vi "configuration UI.vi"() -> ()   [LabVIEW 2013, in "CVT editor node.lvclass"]
uses:
  CVT editor node.lvclass
  <vilib>/CEF_TreeControl/Node/NodeRef.ctl
  <vilib>/CEF_TreeControl/Node/NISE_CEF_Node.lvclass
  <vilib>/NI/AMC/Message Queue.ctl
  <vilib>/NI/AMC/Message.ctl
  <vilib>/NI/Tools/Keyed Array/KeyedArray.ctl
  <vilib>/CEF_TreeControl/Node/UserEventRef.ctl
  <vilib>/CEF_TreeControl/Controls/EventCluster.ctl
  <vilib>/NI/Tag Bus Data Framework/Configuration Editor/Classes/Engine Parent/Engine Parent Editor Node.lvclass
  <vilib>/NI/Tag Bus/tag/tag descriptor.lvclass
  <vilib>/NI/Tag Bus/tag/Data Type.ctl
  <vilib>/NI/TBM Modules/CVT Access/module/configuration/CVT configuration.lvclass
  <vilib>/NI/Module Execution Interface/Engine Configuration/engine configuration.lvclass
  <vilib>/NI/Tag Bus/tag/tag descriptor.lvclass/tag descriptor.ctl
  CVT editor node.lvclass/CVT editor node.ctl
  <vilib>/NI/Tag Bus Module Framework/channel/channel classification.ctl
  <vilib>/NI/Tag Bus Module Framework/root configuration/TBM configuration.lvclass/TBM configuration.ctl
  <vilib>/NI/Tag Bus/tag/write tag name.vi
  <vilib>/NI/Tag Bus/tag/write data type.vi
  <vilib>/NI/Tag Bus Module Framework/root configuration/create GUID.vi
  <vilib>/NI/Tag Bus Data Framework/Configuration Editor/Classes/Module editor node/module editor node.lvclass
  <vilib>/CEF_TreeControl/NISE_CEF_TreeControl.lvlib
  <vilib>/NI/Tag Bus Module Framework/channel/TBM channel.lvclass
  <vilib>/NI/Tag Bus Module Framework/root configuration/TBM configuration.lvclass
  <vilib>/NI/Tools/Keyed Array/Tools_KeyedArray.lvlib
  <vilib>/NI/AMC/AMC.lvlib
panel:
  in  "Tab Control":enum32{"Channel Mapping"}(tab)
  in  "Direction":enum32{"From CVT", "To CVT"}(radio)
  in  "remove to":bool
  in  "add to":bool
  in  "remove from":bool
  in  "add from":bool
  in  "toCVTlist":i32(listbox)
  in  "fromCVTlist":i32(listbox)
  in  "avail tags":i32(listbox)=-1
  in  "user event":T1
  in  "main queue":T2
  in  "node ref":T3
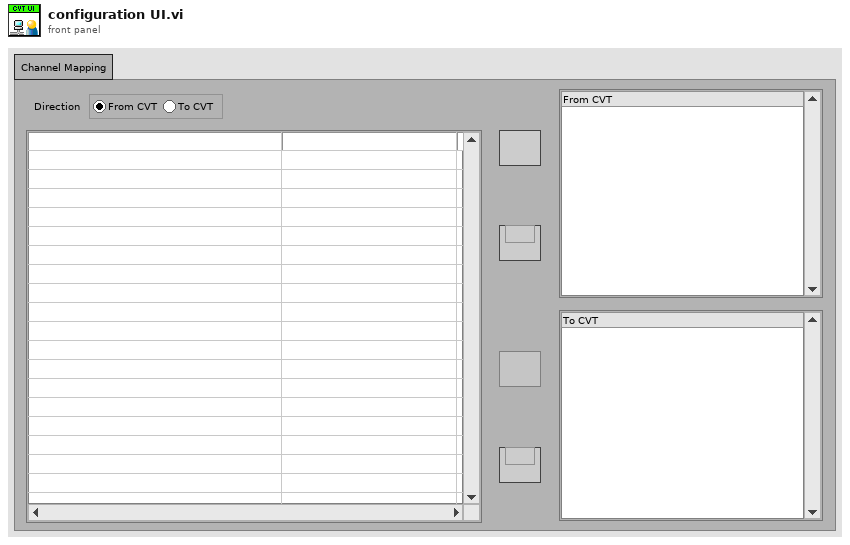
[diagram p1: front panel]
types:
  T1 = typedef "NISE_CEF_Node.lvclass/UserEventRef.ctl" = refnum<user-event>
  T2 = typedef "AMC.lvlib/Message Queue.ctl" = refnum<queue>
  T3 = typedef "NISE_CEF_Node.lvclass/NodeRef.ctl" = refnum<data-value>
  T4 = typedef "NISE_CEF_TreeControl.lvlib/EventCluster.ctl" = cluster{"command":string, "data":string}
  T5 = typedef "tag bus.lvlib/tag descriptor.lvclass/Data Type.ctl" = enum16{"Double", "Single", "I64", "I32", "I16", "I8", "U64", "U32", "U16", "U8", "Boolean", "String", "Array of Double", "Array of Single", "Array of I64", "Array of I32", "Array of I16", "Array of I8", "Array of U64", "Array of U32", "Array of U16", "Array of U8", "Array of Boolean", "Array of String"}
  T6 = enum8{"Enabled", "Disabled", "Disabled and Grayed Out"}
  T7 = typedef "TBM channel.lvclass/channel classification.ctl" = enum16{"input data", "output data", "processing parameter", "processing result"}
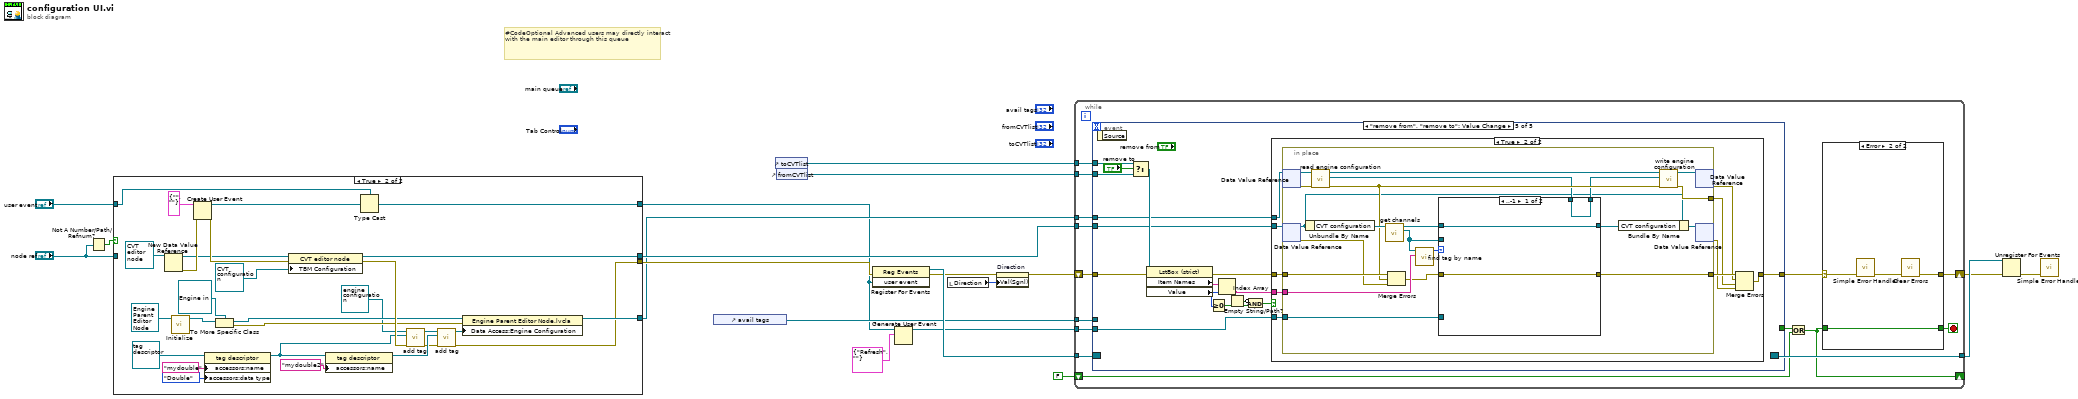
[diagram p0: block diagram]
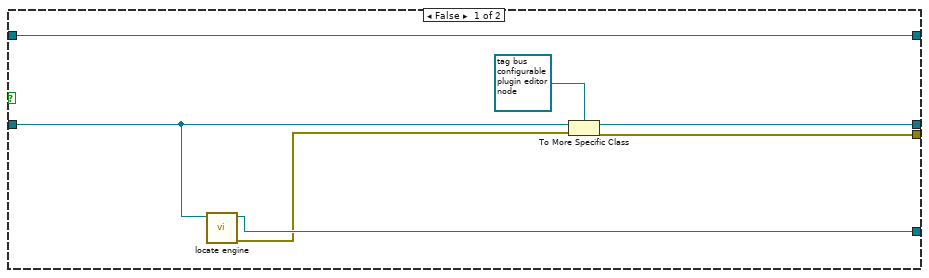
[diagram p2: hidden frame]
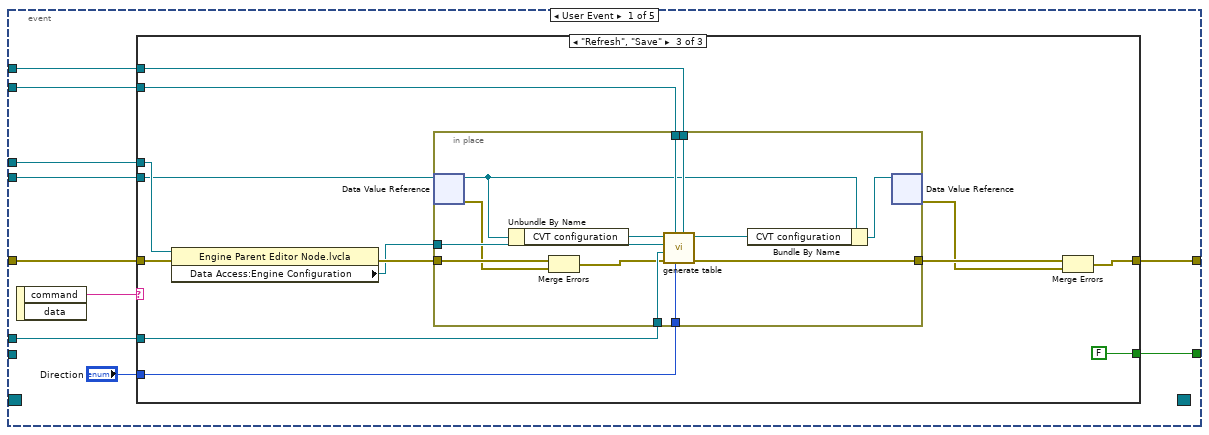
[diagram p4: hidden frame]
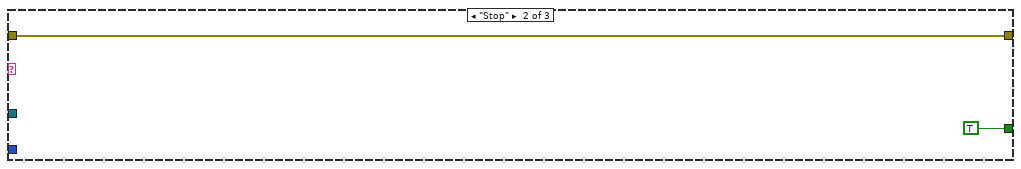
[diagram p6: hidden frame]
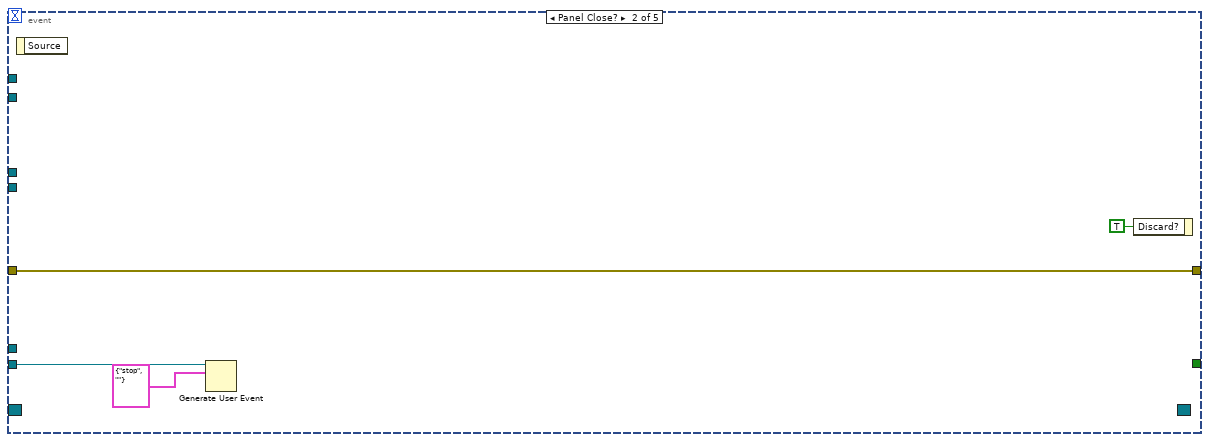
[diagram p7: hidden frame]
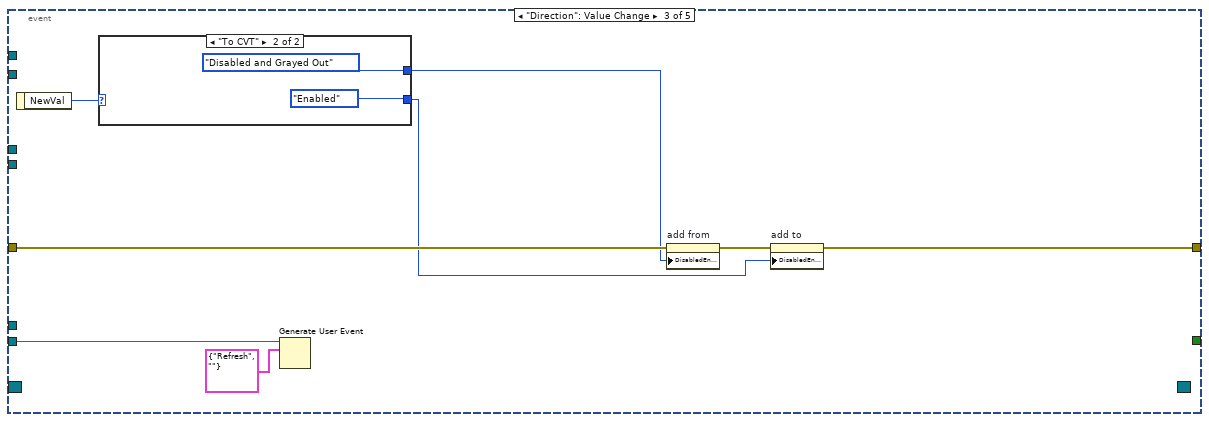
[diagram p8: hidden frame]
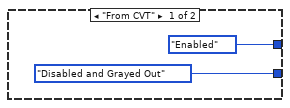
[diagram p9: hidden frame]
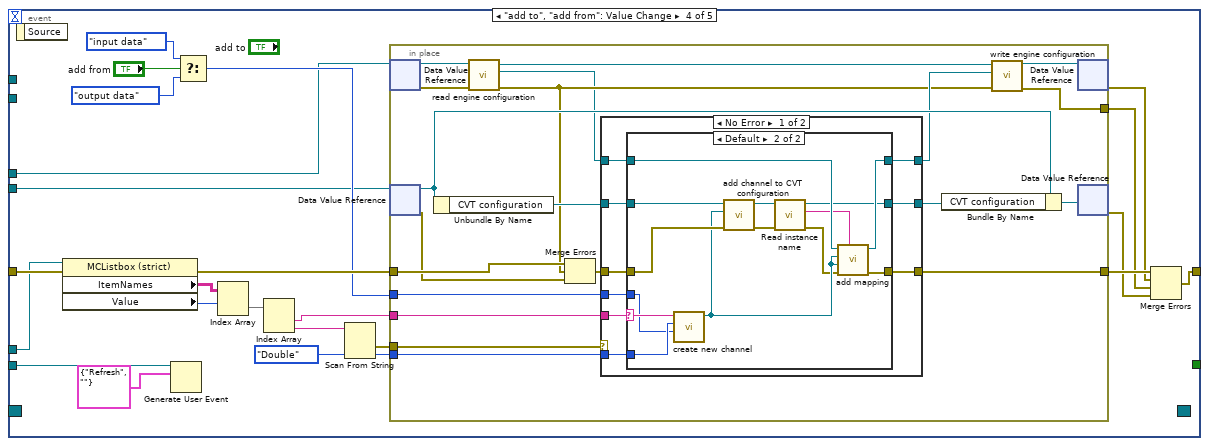
[diagram p10: hidden frame]
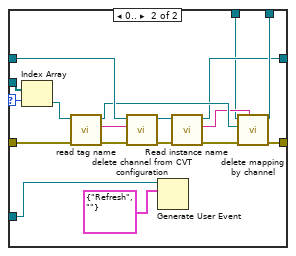
[diagram p14: hidden frame]
diagram:
  # "#CodeOptional Advanced users may directly interact with the main editor through this queue"
  n1 = Not A Number/Path/Refnum?(number/path/refnum="node ref") -> (NaN/Path/Refnum?=w16:bool)
  n2 = case shown="True" w16 {
    tunnel: "user event" -> [w27 w32]
    tunnel: [w27 w33] -> w1
    tunnel: "node ref" -> [w25 _]
    tunnel: [w24 w51] -> w13
    tunnel: [w23 w42] -> w12
    tunnel: [w22 w48] -> w10
    frame False {
      n3 = call <vilib>:"locate engine.vi"("component"=w25) -> ("error out"=w21:errorcluster, "engine"=w22:refnum<data-value>)  [unwired: 9 in]
      n4 = To More Specific Class(target class=refnum<data-value> refnum ("data value reference"), reference=w25, error in=w21) -> (specific class reference=w24:refnum<data-value>, error out=w23:errorcluster)
    }
    frame True {
      n5 = New Data Value Reference(data value=refnum<class "CVT editor node.lvclass"> refnum ("tag bus configurable plugin editor node")) -> (data value reference=w50:refnum<data-value>, error out=w53:errorcluster)  [unwired: 1 in]
      n6 = call-dynamic "Initialize.vi"("Engine in"=refnum<class "Engine Parent Editor Node.lvclass"> refnum) -> ("data value reference"=w37:T3)  [unwired: 8 in, 2 out]
      n7 = Create User Event(user event datatype=T4 {"command"="", "data"=""} ("event data"), error in=w53) -> (user event=w54:refnum<user-event>, error out=w52:errorcluster)
      n8 = property class="tag descriptor"(reference=refnum<class "tag descriptor.lvclass"> refnum ("tag descriptor"), "accessors:name"="mydouble" ("name"), "accessors:data type"=Data_Type."Double" ("data type")) -> (reference out=w40:refnum<class "tag descriptor.lvclass">)  [unwired: 1 in, 1 out]
      n9 = To More Specific Class(target class=refnum<data-value> refnum ("data value reference"), reference=w37) -> (specific class reference=w36:refnum<data-value>, error out=w34:errorcluster)  [unwired: 1 in]
      n10 = property class="CVT editor node"(reference=w50, error in=w52, "TBM Configuration"=refnum<class "CVT configuration.lvclass"> refnum ("CVT configuration")) -> (reference out=w51:refnum<data-value>, error out=w44:errorcluster)
      n11 = property class="tag descriptor"(reference=w40, "accessors:name"="mydouble2" ("name")) -> (reference out=w41:refnum<class "tag descriptor.lvclass">)  [unwired: 1 in, 1 out]
      n12 = Type Cast(type=w32, x=w54) -> (*(type *) &x=w33:T1)
      n13 = call <vilib>:"add tag.vi"("error in"=w44, "tag descriptor"=w40, "engine configuration in"=refnum<class "engine configuration.lvclass"> refnum) -> ("error out"=w31:errorcluster, "engine configuration out"=w30:refnum<class "engine configuration.lvclass">)  [unwired: 7 in]
      n14 = call <vilib>:"add tag.vi"("error in"=w31, "tag descriptor"=w41, "engine configuration in"=w30) -> ("error out"=w42:errorcluster, "engine configuration out"=w29:refnum<class "engine configuration.lvclass">)  [unwired: 7 in]
      n15 = property class="Engine Parent Editor Node.lvcla"(reference=w36, error in=w34, "Data Access:Engine Configuration"=w29) -> (reference out=w48:refnum<data-value>)  [unwired: 1 out]
    }
  }
  n16 = control-ref of="avail tags"() -> (w9:refnum<vi>)
  n17 = control-ref of="toCVTlist"() -> (w8:refnum<vi>)
  n18 = control-ref of="fromCVTlist"() -> (w7:refnum<vi>)
  n19 = register-events(error in=w12, w1) -> (reference out=w20:refnum<event-registration>, error out=w6:errorcluster)  [unwired: 1 in]
  n20 = Generate User Event(user event=w1, event data cluster=T4 {"command"="Refresh", "data"=""} ("event data")) -> (user event out=w2:T1)  [unwired: 2 in, 1 out]
  n21 = local read "Direction"() -> (w4:enum32{"From CVT", "To CVT"})
  n22 = property on="Direction" class="RadioBtnsControl (strict)"(error in=w6, "Val(Sgnl)"=w4) -> (error out=w5:errorcluster)  [unwired: 1 in, 1 out]
  n23 = while {
    tunnel: w20 -> [w70]
    tunnel: [w69] -> w19
    shift-right: [w62] -> w18
    shift-left: w5 -> [w68]
    shift-right: [w64] -> _
    shift-left: FALSE -> [w63]
    tunnel: w13 -> [w61]
    tunnel: w10 -> [w60]
    tunnel: w2 -> [w59]
    tunnel: w9 -> [w58]
    tunnel: w8 -> [w57]
    tunnel: w7 -> [w56]
    stop <- w66 stop-if-true
    n24 = event shown="[4] \"remove from\", \"remove to\": Value Change" {
      selector: w70 -> [_ _ _ _ _]
      dyn-events: [_ _ _ _ _] -> w69
      timeout: _ -> [_ _ _ _ _]
      tunnel: [w86 _ _ _ _] -> w65
      tunnel: [w83 w119 w123 w137 w209] -> w67
      tunnel: w68 -> [w84 w119 w125 w155 w217]
      tunnel: w61 -> [w82 _ _ w133 w206]
      tunnel: w60 -> [w81 _ _ w134 w205]
      tunnel: w59 -> [_ w116 w126 w153 w208]
      tunnel: w58 -> [w80 _ _ w147 _]
      tunnel: w57 -> [w79 _ _ _ w219]
      tunnel: w56 -> [w78 _ _ _ w220]
      event User Event {
        n25 = event-data() -> ("command"=w85:string)  [unwired: 1 in, 1 out]
        n26 = case shown="\"Refresh\", \"Save\"" w85 {
          tunnel: [_ TRUE FALSE] -> w86
          tunnel: w84 -> [w87 w88 w101]
          tunnel: [w87 w88 w91] -> w83
          tunnel: w82 -> [_ _ w92]
          tunnel: w81 -> [_ _ w94]
          tunnel: w80 -> [_ _ w99]
          tunnel: w79 -> [_ _ w98]
          tunnel: w78 -> [_ _ w97]
          tunnel: "Direction" -> [_ _ w96]
          frame Default {
          }
          frame "Stop" {
          }
          frame "Refresh", "Save" {
            n27 = property class="Engine Parent Editor Node.lvcla"(reference=w94, error in=w101) -> (error out=w95:errorcluster, "Data Access:Engine Configuration"=w93:refnum<class "engine configuration.lvclass">)  [unwired: 1 out]
            n28 = in-place {
              in-place-border: [w115] -> w100
              in-place-border: w99 -> [w114]
              in-place-border: w98 -> [w113]
              in-place-border: w97 -> [w112]
              in-place-border: w96 -> [w111]
              in-place-border: w95 -> [w110]
              in-place-border: w93 -> [w109]
              n29 = in-place-dvr #1(w92) -> (w105:refnum<class "CVT editor node.lvclass">, w107:errorcluster)
              n30 = Unbundle By Name(w105) -> ("CVT configuration"=w106:refnum<class "CVT configuration.lvclass">)
              n31 = Merge Errors(w110, w107) -> (w108:errorcluster)
              n32 = call "generate table.vi"("to cvt"=w113, "Direction"=w111, "from cvt"=w112, "error in"=w108, "avail tags"=w114, "engine configuration in"=w109, "cvt in"=w106) -> ("error out"=w115:errorcluster, "cvt out"=w103:refnum<class "CVT configuration.lvclass">)  [unwired: 3 in]
              n33 = Bundle By Name(cluster=w105, "CVT configuration"=w103) -> (w104:refnum<class "CVT editor node.lvclass">)
              n34 = in-place-dvr #1(w104) -> (w90:errorcluster)  [unwired: 1 out]
            }
            n35 = Merge Errors(w100, w90) -> (w91:errorcluster)
          }
        }
      }
      event Panel Close? {
        n36 = event-data() -> ()  [unwired: 1 in, 1 out]
        n37 = Generate User Event(user event=w116, event data cluster=T4 {"command"="stop", "data"=""} ("event data")) -> ()  [unwired: 2 in, 2 out]
        n38 = event-data("Discard?"=TRUE) -> ()  [unwired: 1 in, 1 out]
      }
      event "Direction": Value Change {
        n39 = event-data() -> ("NewVal"=w122:enum32{"From CVT", "To CVT"})  [unwired: 1 in]
        n40 = case shown="\"To CVT\"" w122 {
          tunnel: [T6."Enabled" ("Disabled") T6."Disabled and Grayed Out" ("Disabled")] -> w121
          tunnel: [T6."Disabled and Grayed Out" ("Disabled") T6."Enabled" ("Disabled")] -> w120
          frame "From CVT" {
          }
          frame "To CVT" {
          }
        }
        n41 = Generate User Event(user event=w126, event data cluster=T4 {"command"="Refresh", "data"=""} ("event data")) -> ()  [unwired: 2 in, 2 out]
        n42 = property on="add from" class="Bool"(error in=w125, "DisabledEnum"=w121) -> (error out=w124:errorcluster)  [unwired: 1 in, 1 out]
        n43 = property on="add to" class="Bool"(error in=w124, "DisabledEnum"=w120) -> (error out=w123:errorcluster)  [unwired: 1 in, 1 out]
      }
      event "add to", "add from": Value Change {
        n44 = event-data() -> ()  [unwired: 1 in, 1 out]
        n45 = property class="MCListbox (strict)"(reference=w147, error in=w155) -> (error out=w148:errorcluster, "ItemNames"=w146:string[][], "Value"=w145:i32)  [unwired: 1 out]
        n46 = Generate User Event(user event=w153, event data cluster=T4 {"command"="Refresh", "data"=""} ("event data")) -> ()  [unwired: 2 in, 2 out]
        n47 = Select(t=channel_classification."input data" ("channel classification"), s="add from", f=channel_classification."output data" ("channel classification")) -> (s? t:f=w138:T7)
        n48 = Index Array(array=w146, index (row)=w145) -> (element=w142:string[])  [unwired: 1 in]
        n49 = Index Array(array=w142) -> (element #1=w141:string, element #2=w144:string)  [unwired: 2 in]
        n50 = Scan From String(input string=w144, default 1=Data_Type."Double" ("data type")) -> (error out=w140:errorcluster, output 1=w139:T5)  [unwired: 3 in, 2 out]
        n51 = in-place {
          in-place-border: [w175] -> w154
          in-place-border: w148 -> [w174]
          in-place-border: w141 -> [w173]
          in-place-border: w140 -> [w172]
          in-place-border: w139 -> [w171]
          in-place-border: w138 -> [w170]
          in-place-border: [w160] -> w132
          n52 = in-place-dvr #2(w134) -> (w163:refnum<class "Engine Parent Editor Node.lvclass">, w158:errorcluster)
          n53 = in-place-dvr #3(w133) -> (w166:refnum<class "CVT editor node.lvclass">, w164:errorcluster)
          n54 = Unbundle By Name(w166) -> ("CVT configuration"=w168:refnum<class "CVT configuration.lvclass">)
          n55 = call <vilib>:"read engine configuration.vi"("error in"=w158, "Engine Parent Editor Node in"=w163) -> ("error out"=w157:errorcluster, "engine configuration"=w156:refnum<class "engine configuration.lvclass">, "Engine Parent Editor Node out"=w159:refnum<class "Engine Parent Editor Node.lvclass">)  [unwired: 7 in]
          n56 = Merge Errors(w174, w157, w164) -> (w169:errorcluster)
          n57 = case shown="No Error" w172 {
            tunnel: [w184 w202] -> w175
            tunnel: [w183 w204] -> w161
            tunnel: [w182 w203] -> w167
            tunnel: w168 -> [w181 w203]
            tunnel: w156 -> [w180 w204]
            tunnel: w169 -> [w179 w202]
            tunnel: w173 -> [w178 _]
            tunnel: w171 -> [w177 _]
            tunnel: w170 -> [w176 _]
            frame No Error {
              n58 = case shown="Default" w178 {
                selector: w178 -> [_ w195]
                tunnel: [w187 w201] -> w184
                tunnel: w179 -> [w187 w197]
                tunnel: w180 -> [w185 w200]
                tunnel: [w186 w189] -> w182
                tunnel: w181 -> [w186 w198]
                tunnel: [w185 w199] -> w183
                tunnel: w177 -> [_ w194]
                tunnel: w176 -> [_ w193]
                frame "" {
                }
                frame Default {
                  n59 = call <vilib>:"create new channel.vi"("channel classification"=w193, "data type"=w194, "channel name"=w195) -> ("channel"=w192:refnum<class "TBM channel.lvclass">)  [unwired: 8 in]
                  n60 = call <vilib>:"add channel to CVT configuration.vi"("error in"=w197, "channel"=w192, "CVT configuration in"=w198) -> ("error out"=w196:errorcluster, "CVT configuration out"=w190:refnum<class "CVT configuration.lvclass">)  [unwired: 7 in]
                  n61 = call <vilib>:"Read instance name.vi"("error in"=w196, "configuration in"=w190) -> ("error out"=w191:errorcluster, "instance id"=w188:string, "configuration out"=w189:refnum<class "CVT configuration.lvclass">)  [unwired: 7 in]
                  n62 = call <vilib>:"add mapping.vi"("owner ID"=w188, "error in"=w191, "channel"=w192, "tag descriptor"=w192, "engine configuration"=w200) -> ("error out"=w201:errorcluster, "engine configuration out"=w199:refnum<class "engine configuration.lvclass">)  [unwired: 5 in]
                }
              }
            }
            frame Error {
            }
          }
          n63 = Bundle By Name(cluster=w166, "CVT configuration"=w167) -> (w165:refnum<class "CVT editor node.lvclass">)
          n64 = call <vilib>:"write engine configuration.vi"("error in"=w157, "engine configuration"=w161, "Engine Parent Editor Node in"=w159) -> ("error out"=w160:errorcluster, "Engine Parent Editor Node out"=w162:refnum<class "Engine Parent Editor Node.lvclass">)  [unwired: 7 in]
          n65 = in-place-dvr #2(w162) -> (w136:errorcluster)  [unwired: 1 out]
          n66 = in-place-dvr #3(w165) -> (w135:errorcluster)  [unwired: 1 out]
        }
        n67 = Merge Errors(w154, w136, w132, w135) -> (w137:errorcluster)
      }
      event "remove from", "remove to": Value Change {
        n68 = event-data() -> ()  [unwired: 1 in, 1 out]
        n69 = Select(t=w219, s="remove to", f=w220) -> (s? t:f=w216:refnum<vi>)
        n70 = property class="LstBox (strict)"(reference=w216, error in=w217) -> (error out=w210:errorcluster, "Item Names"=w215:string[], "Value"=w214:i32)  [unwired: 1 out]
        n71 = Greater Or Equal To 0?(x=w214) -> (x >= 0?=w212:bool)
        n72 = Index Array(array=w215, index=w214) -> (element=w207:string)
        n73 = Empty String/Path?(string/path=w207) -> (empty?=w213:bool)
        n74 = Compound Arithmetic op=AND(invert w213, w212) -> (w211:bool)
        n75 = case shown="True" w211 {
          tunnel: w210 -> [w221 w228]
          tunnel: [w221 w227] -> w209
          tunnel: w208 -> [_ w231]
          tunnel: w207 -> [_ w230]
          tunnel: w206 -> [_ w226]
          tunnel: w205 -> [_ w225]
          frame False {
          }
          frame True {
            n76 = in-place {
              in-place-border: w231 -> [w252]
              in-place-border: w230 -> [w251]
              in-place-border: [w248] -> w229
              in-place-border: w228 -> [w247]
              in-place-border: [w241] -> w222
              n77 = in-place-dvr #4(w225) -> (w244:refnum<class "Engine Parent Editor Node.lvclass">, w239:errorcluster)
              n78 = in-place-dvr #5(w226) -> (w234:refnum<class "CVT editor node.lvclass">, w238:errorcluster)
              n79 = Unbundle By Name(w234) -> ("CVT configuration"=w240:refnum<class "CVT configuration.lvclass">)
              n80 = call <vilib>:"read engine configuration.vi"("error in"=w239, "Engine Parent Editor Node in"=w244) -> ("error out"=w237:errorcluster, "engine configuration"=w236:refnum<class "engine configuration.lvclass">, "Engine Parent Editor Node out"=w243:refnum<class "Engine Parent Editor Node.lvclass">)  [unwired: 7 in]
              n81 = call-dynamic "get channels.vi"("CVT configuration in"=w240) -> ("channels"=w246:refnum<class "TBM channel.lvclass">[], "CVT configuration out"=w249:refnum<class "CVT configuration.lvclass">)  [unwired: 9 in]
              n82 = Merge Errors(w247, w237, w238) -> (w245:errorcluster)
              n83 = call <vilib>:"find tag by name.vi"("name"=w251, "tags in"=w246) -> ("index"=w250:i32)  [unwired: 9 in]
              n84 = case shown="..-1" w250 {
                selector: w250 -> [_ w271]
                tunnel: w252 -> [_ w272]
                tunnel: w249 -> [w255 w269]
                tunnel: [w255 w258] -> w232
                tunnel: [w254 w265] -> w248
                tunnel: w245 -> [w254 w268]
                tunnel: [w253 w266] -> w235
                tunnel: w246 -> [_ w270]
                tunnel: w236 -> [w253 w256]
                frame ..-1 {
                }
                frame 0.. {
                  n85 = Index Array(array=w270, index=w271) -> (element=w263:refnum<class "TBM channel.lvclass">)
                  n86 = call <vilib>:"read tag name.vi"("error in"=w268, "system tag in"=w263) -> ("error out"=w264:errorcluster, "name"=w261:string, "system tag out"=w262:refnum<class "TBM channel.lvclass">)  [unwired: 7 in]
                  n87 = call <vilib>:"delete channel from CVT configuration.vi"("error in"=w264, "channel to delete"=w261, "CVT configuration in"=w269) -> ("error out"=w267:errorcluster, "CVT configuration out"=w259:refnum<class "CVT configuration.lvclass">)  [unwired: 7 in]
                  n88 = Generate User Event(user event=w272, event data cluster=T4 {"command"="Refresh", "data"=""} ("event data")) -> ()  [unwired: 2 in, 2 out]
                  n89 = call <vilib>:"Read instance name.vi"("error in"=w267, "configuration in"=w259) -> ("error out"=w260:errorcluster, "instance id"=w257:string, "configuration out"=w258:refnum<class "CVT configuration.lvclass">)  [unwired: 7 in]
                  n90 = call <vilib>:"delete mapping by channel.vi"("owner ID"=w257, "error in"=w260, "channel"=w262, "engine configuration in"=w256) -> ("error out"=w265:errorcluster, "engine configuration out"=w266:refnum<class "engine configuration.lvclass">)  [unwired: 6 in]
                }
              }
              n91 = Bundle By Name(cluster=w234, "CVT configuration"=w232) -> (w233:refnum<class "CVT editor node.lvclass">)
              n92 = call <vilib>:"write engine configuration.vi"("error in"=w237, "engine configuration"=w235, "Engine Parent Editor Node in"=w243) -> ("error out"=w241:errorcluster, "Engine Parent Editor Node out"=w242:refnum<class "Engine Parent Editor Node.lvclass">)  [unwired: 7 in]
              n93 = in-place-dvr #4(w242) -> (w224:errorcluster)  [unwired: 1 out]
              n94 = in-place-dvr #5(w233) -> (w223:errorcluster)  [unwired: 1 out]
            }
            n95 = Merge Errors(w229, w224, w222, w223) -> (w227:errorcluster)
          }
        }
      }
    }
    n96 = Or(x=w65, y=w63) -> (x .or. y?=w64:bool)
    n97 = case shown="Error" w67 {
      selector: w67 -> [w71 w75]
      tunnel: [w72 w76] -> w66
      tunnel: w64 -> [w72 w76]
      tunnel: [w71 w73] -> w62
      frame No Error {
      }
      frame Error {
        n98 = call <vilib>:"Simple Error Handler.vi"("error in (no error)"=w75) -> ("error out"=w74:errorcluster)  [unwired: 4 in, 4 out]
        n99 = call <vilib>:"Clear Errors.vi"("error in (no error)"=w74) -> ("error out"=w73:errorcluster)  [unwired: 6 in]
      }
    }
  }
  n100 = Unregister For Events(event registration refnum=w19, error in=w18) -> (error out=w11:errorcluster)
  n101 = call <vilib>:"Simple Error Handler.vi"("error in (no error)"=w11) -> ()  [unwired: 4 in, 5 out]
